vi "PowerSuppliesControlVoltageMode.vi"(4 "Z-":dbl, 5 "OnOff":bool, 6 "Z+":dbl, 7 "Max Voltage (V)":dbl=1.0, 8 "Y-":dbl, 9 "Y+":dbl, 10 "X-":dbl, 11 "X+":dbl) -> (3 "Saturating":bool)   [LabVIEW 2020]
uses:
  <vilib>/imath/engines/lvmath2/RunTimeEngine/Managers/WorkSpace/UID Generator.vi
  <vilib>/imath/engines/lvmath2/RunTimeEngine/BuiltInFunctions/abs/NIMS_abs(signed).vi
  <instcachedir>/0/NIMS_abs(signed)_C4FCB8E6058B49B797C7C8D53CA5F6EC.lvgen/NIMS_abs(signed)_C4FCB8E6058B49B797C7C8D53CA5F6EC_001.vi
  <vilib>/imath/engines/lvmath2/RunTimeEngine/BuiltInFunctions/max/1 input/NIMS_max(RV).vi
  <instcachedir>/0/NIMS_max(RV)_237633DB1D604D5BA7001287DF3C7957.lvgen/NIMS_max(RV)_237633DB1D604D5BA7001287DF3C7957_000.vi
  <vilib>/imath/engines/lvmath2/RunTimeEngine/RunTimeType/NIMS_RunTimeType_From StrictType (excl LVString).vi
  <instcachedir>/0/NIMS_RunTimeType_From StrictType (excl LVString)_283B1B2000484AAA8744D21CE97EA49F.lvgen/NIMS_RunTimeType_From StrictType (excl LVString)_283B1B2000484AAA8744D21CE97EA49F_000.vi
  <vilib>/imath/engines/lvmath2/RunTimeEngine/LocalVariableDefStatement/MC_LocalVariableDefStatement_Display.vi
  <vilib>/imath/engines/lvmath2/RunTimeEngine/RunTimeType/NIMS_RunTimeType_Set Source Original Bool.vi
  <vilib>/imath/engines/lvmath2/RunTimeEngine/IndexRead/NIMS V(S).vi
  <instcachedir>/0/NIMS V(S)_0488751826AF41519A22953C041130DC.lvgen/NIMS V(S)_0488751826AF41519A22953C041130DC_000.vi
  <vilib>/imathl/engines/lvmath/Functions/Error Handling/Create Error.vi
  <vilib>/imath/engines/lvmath2/RunTimeEngine/Managers/SymbolTable/Clear UID.vi
  <vilib>/imath/engines/lvmath2/RunTimeEngine/NodeEndStatement/NIMS_NodeEndStatement_Output.vi
  <instcachedir>/0/NIMS_NodeEndStatement_Output_53EC0D466D134D7ABD903AC30B43404B.lvgen/NIMS_NodeEndStatement_Output_53EC0D466D134D7ABD903AC30B43404B_010.vi
  <instcachedir>/0/NIMS_NodeEndStatement_Output_53EC0D466D134D7ABD903AC30B43404B.lvgen/NIMS_NodeEndStatement_Output_53EC0D466D134D7ABD903AC30B43404B_001.vi
  <vilib>/imath/engines/lvmath2/RunTimeEngine/ErrorHandling/NIMS_Finalize Error.vi
  <vilib>/imath/engines/lvmath2/RunTimeEngine/Managers/SymbolTable/NIMS_WorkSpace.lvlib
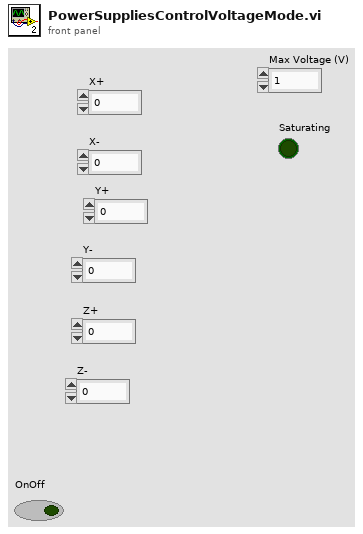
[diagram p1: front panel]
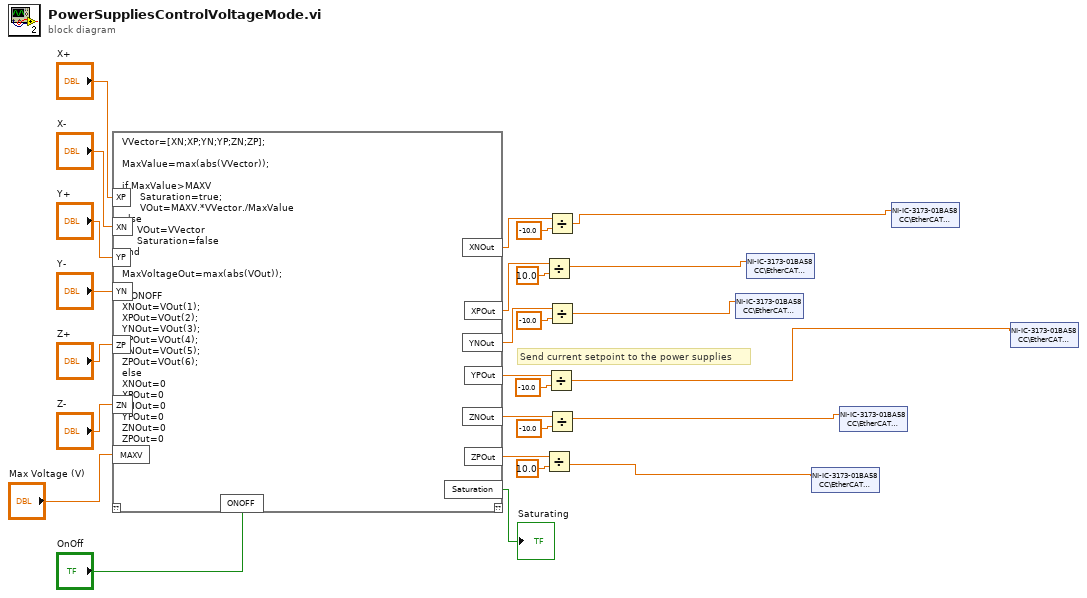
[diagram p0: block diagram]
diagram:
  # "Send current setpoint to the power supplies"
  n1 = mathscript code="VVector=[XN;XP;YN;YP;ZN;ZP];\n\nMaxValue=max(abs(VVector));\n\nif MaxValue>MAXV\n      Saturation=true;\n      VOut=MAXV.*VVector./MaxValue\nelse\n     VOut=VVector\n     Saturation=false\nend\n\nMaxVoltageOut=max(abs(VOut));\n\nif ONOFF\nXNOut=VOut(1);\nXPOut=VOut(2);\nYNOut=VOut(3);\nYPOut=VOut(4);\nZNOut=VOut(5);\nZPOut=VOut(6);\nelse\nXNOut=0\nXPOut=0\nYNOut=0\nYPOut=0\nZNOut=0\nZPOut=0\nend"("YP"="Y+", "YN"="Y-", "XP"="X+", "XN"="X-", "ZP"="Z+", "ZN"="Z-", "MAXV"="Max Voltage (V)", "ONOFF"="OnOff") -> ("XNOut"=w11:dbl, "XPOut"=w13:dbl, "YNOut"=w10:dbl, "YPOut"=w14:dbl, "ZNOut"=w12:dbl, "ZPOut"=w9:dbl, "Saturation"=→"Saturating":bool)  [unwired: 1 in, 1 out]
  n2 = Divide(x=w13, y=10.0) -> (x/y=w5:dbl)
  n3 = Divide(x=w9, y=10.0) -> (x/y=w2:dbl)
  n4 = Divide(x=w14, y=-10.0) -> (x/y=w1:dbl)
  n5 = Divide(x=w11, y=-10.0) -> (x/y=w6:dbl)
  n6 = Divide(x=w10, y=-10.0) -> (x/y=w4:dbl)
  n7 = Divide(x=w12, y=-10.0) -> (x/y=w3:dbl)
  n8 = shared-variable "NI-IC-3173-01BA58CC\\EtherCAT Master\\Device\\Mod1\\AO2"(w4) -> ()  [unwired: 1 in, 1 out]
  n9 = shared-variable "NI-IC-3173-01BA58CC\\EtherCAT Master\\Device\\Mod1\\AO0"(w5) -> ()  [unwired: 1 in, 1 out]
  n10 = shared-variable "NI-IC-3173-01BA58CC\\EtherCAT Master\\Device\\Mod2\\AO1"(w2) -> ()  [unwired: 1 in, 1 out]
  n11 = shared-variable "NI-IC-3173-01BA58CC\\EtherCAT Master\\Device\\Mod1\\AO1"(w3) -> ()  [unwired: 1 in, 1 out]
  n12 = shared-variable "NI-IC-3173-01BA58CC\\EtherCAT Master\\Device\\Mod1\\AO3"(w6) -> ()  [unwired: 1 in, 1 out]
  n13 = shared-variable "NI-IC-3173-01BA58CC\\EtherCAT Master\\Device\\Mod2\\AO0"(w1) -> ()  [unwired: 1 in, 1 out]
